vi "Set Data Replay Component Properties.vi"(8 "error in (no error)":errorcluster, 9 "Prefix#":i32, 10 "DataReplays":T2[](array[typedef]), 11 "Item Ref in":T1 format="%.0x") -> (0 "error out":errorcluster, 3 "Item Ref out":T1 format="%.0x")   [LabVIEW 2011, in "Engine Sim System Explorer.lvlib"]
uses:
  Engine Sim System Explorer.lvlib
  <vilib>/NI Veristand/Custom Device API/Custom Device Item Ref.ctl
  TypeDefs/DataReplayComp.ctl
  Shared/Engine Simulation Global.vi
  <vilib>/NI Veristand/Custom Device API/Set Item Property (I32).vi
  <vilib>/NI Veristand/Custom Device API/Set Item Property (String).vi
  <vilib>/NI Veristand/Custom Device API/Set Item Property (Variant).vi
  <vilib>/NI Veristand/Custom Device API/Custom Device API.lvlib
  Engine Simulation Shared.lvlib
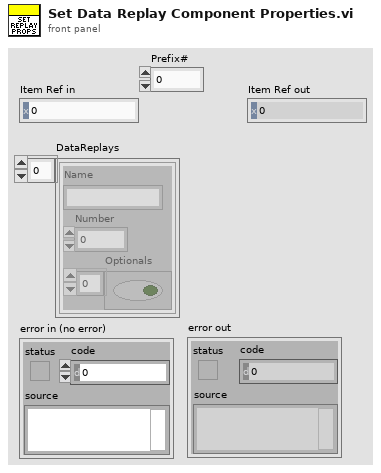
[diagram p1: front panel]
types:
  T1 = typedef "Custom Device API.lvlib/Custom Device Item Ref.ctl" = u64
  T2 = typedef "Engine Sim System Explorer.lvlib/DataReplayComp.ctl" = cluster{"Name":string, "Number":i32, "Optionals":bool[]}
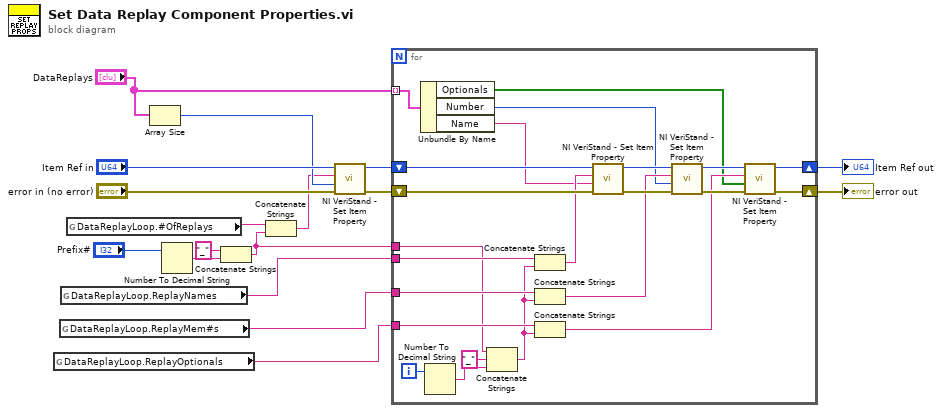
[diagram p0: block diagram]
diagram:
  n1 = global read "Engine Simulation Global.vi" "DataReplayLoop.ReplayOptionals"() -> (w9:string)
  n2 = global read "Engine Simulation Global.vi" "DataReplayLoop.ReplayMem#s"() -> (w10:string)
  n3 = global read "Engine Simulation Global.vi" "DataReplayLoop.ReplayNames"() -> (w11:string)
  n4 = global read "Engine Simulation Global.vi" "DataReplayLoop.#OfReplays"() -> (w3:string)
  n5 = Array Size(array="DataReplays") -> (size(s)=w15:i32)
  n6 = Number To Decimal String(number="Prefix#") -> (decimal integer string=w5:string)  [unwired: 1 in]
  n7 = Concatenate Strings("_" ("string"), w5) -> (w1:string)
  n8 = Concatenate Strings(w3, w1) -> (w2:string)
  n9 = call-poly <vilib>:"NI VeriStand - Set Item Property.vi"("error in (no error)"="error in (no error)", "Value"=w15, "Property Name"=w2, "Item Ref in"="Item Ref in") -> ("error out"=w14:errorcluster, "Item Ref out"=w12:T1)  [unwired: 5 in, 1 out]
  n10 = for {
    shift-right: [w20] -> w8
    shift-left: w14 -> [w32]
    tunnel: "DataReplays" -> [w40] mode=indexing
    shift-right: [w19] -> w7
    shift-left: w12 -> [w31]
    tunnel: w11 -> [w38]
    tunnel: w10 -> [w35]
    tunnel: w9 -> [w34]
    tunnel: w1 -> [w18]
    i -> [w39]
    n11 = Unbundle By Name(w40) -> ("Optionals"=w21:bool[], "Number"=w25:i32, "Name"=w29:string)
    n12 = Number To Decimal String(number=w39) -> (decimal integer string=w37:string)  [unwired: 1 in]
    n13 = Concatenate Strings(w18, "_" ("string"), w37) -> (w33:string)
    n14 = Concatenate Strings(w38, w33) -> (w30:string)
    n15 = Concatenate Strings(w35, w33) -> (w26:string)
    n16 = Concatenate Strings(w34, w33) -> (w22:string)
    n17 = call-poly <vilib>:"NI VeriStand - Set Item Property.vi"("error in (no error)"=w32, "Value"=w29, "Property Name"=w30, "Item Ref in"=w31) -> ("error out"=w28:errorcluster, "Item Ref out"=w27:T1)  [unwired: 5 in, 1 out]
    n18 = call-poly <vilib>:"NI VeriStand - Set Item Property.vi"("error in (no error)"=w28, "Value"=w25, "Property Name"=w26, "Item Ref in"=w27) -> ("error out"=w24:errorcluster, "Item Ref out"=w23:T1)  [unwired: 5 in, 1 out]
    n19 = call-poly <vilib>:"NI VeriStand - Set Item Property.vi"("error in (no error)"=w24, "Value"=w21, "Property Name"=w22, "Item Ref in"=w23) -> ("error out"=w20:errorcluster, "Item Ref out"=w19:T1)  [unwired: 5 in, 1 out]
  }
  "error out" <- w8
  "Item Ref out" <- w7
